vi "FTW-JSON-ObjectManip-AddPair.vi"(0 "Input JSON Object":string, 5 "Key":string, 7 "Value":string, 11 "error in":errorcluster) -> (4 "Output JSON Object":string, 15 "error out":errorcluster)   [LabVIEW 2015]
uses:
  container/FTW-Container.lvclass
panel:
  # "Inputs"
  # "Outputs"
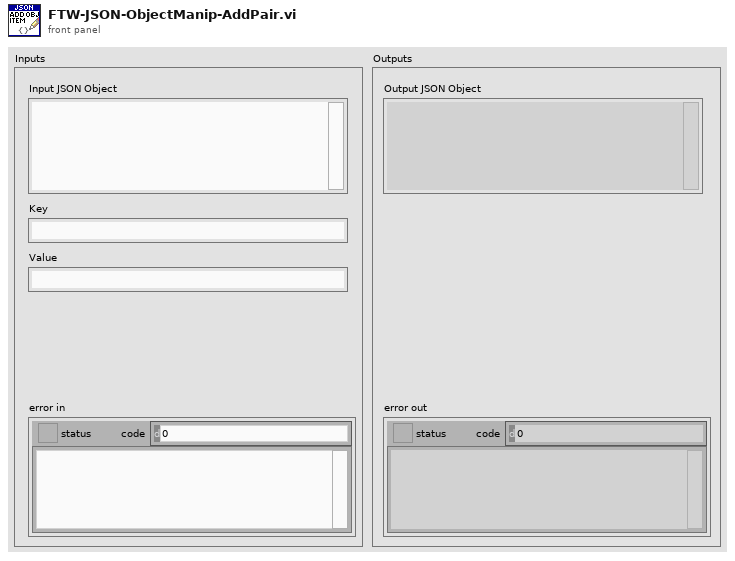
[diagram p1: front panel]
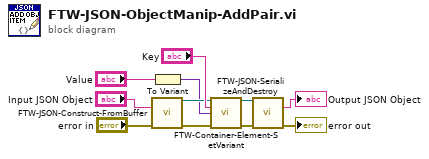
[diagram p0: block diagram]
diagram:
  n1 = call "FTW-JSON-Construct-FromBuffer.vi"("JSON String (UTF-8)"="Input JSON Object", "error in"="error in") -> ("JSON"=w6:refnum<class "FTW-Container.lvclass">, "error out"=w4:errorcluster)  [unwired: 12 in]
  n2 = To Variant(anything="Value") -> (Variant=w1:variant)
  n3 = call "FTW-Container-Element-SetVariant.vi"("FTW-Container In"=w6, "Element Name"="Key", "Variant"=w1, "error in"=w4) -> ("FTW-Container Out"=w5:refnum<class "FTW-Container.lvclass">, "error out"=w3:errorcluster)  [unwired: 9 in, 1 out]
  n4 = call "FTW-JSON-SerializeAndDestroy.vi"("JSON"=w5, "error in"=w3) -> ("JSON String (UTF-8)"=→"Output JSON Object":string, "error out"=→"error out":errorcluster)  [unwired: 12 in]
